vi "upload.list_parts.vi"(8 "error in":errorcluster, 11 "Multipart Upload":refnum<class "Multipart Upload.lvclass">) -> (0 "error out":errorcluster, 3 "Multipart Upload out":refnum<class "Multipart Upload.lvclass">)   [LabVIEW 2020, in "Multipart Upload.lvclass"]
doc: "Lists the parts that have been uploaded for a given uploadId."
uses:
  Multipart Upload.lvclass
  Multipart Upload.lvclass/Multipart Upload.ctl
  Nominal Client/Nominal Client.lvclass/Nominal Client.ctl
  72e5dcd8-64cf-4027-aada-cf32ea863567.vi
  nominal_client.get.vi
  parts.set.vi
  Nominal Client/create.authorization_header.vi
  Nominal Client/trace.payload_sent.vi
  Nominal Client/trace.payload_received.vi
  Nominal Client/error.vi
  Nominal Client/api_token.get.vi
  Nominal Client/error.vi/859f8e04-e495-489b-b5b4-7ac163f56130.vi
  submodules/reqwest-labview/lv-src/reqwest/get.vi
  <vilib>/JDP Science/JSONtext/Get all Object Items.vi
  <vilib>/Utility/error.llb/Error Cluster From Error Code.vi
  <vilib>/JDP Science/JSONtext/JSON text to Variant.vi
  Nominal Client/Nominal Client.lvclass
  <vilib>/JDP Science/JSONtext/LVClass Serializer/JSONtext LVClass Serializer.lvclass
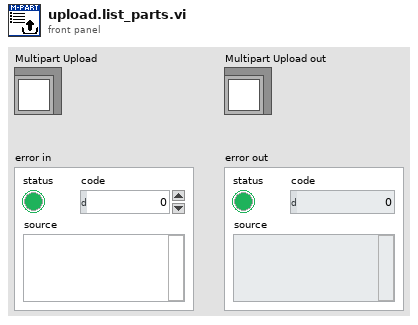
[diagram p1: front panel]
types:
  T1 = cluster{"partNumber":i32, "etag":string, "size":i32}[]
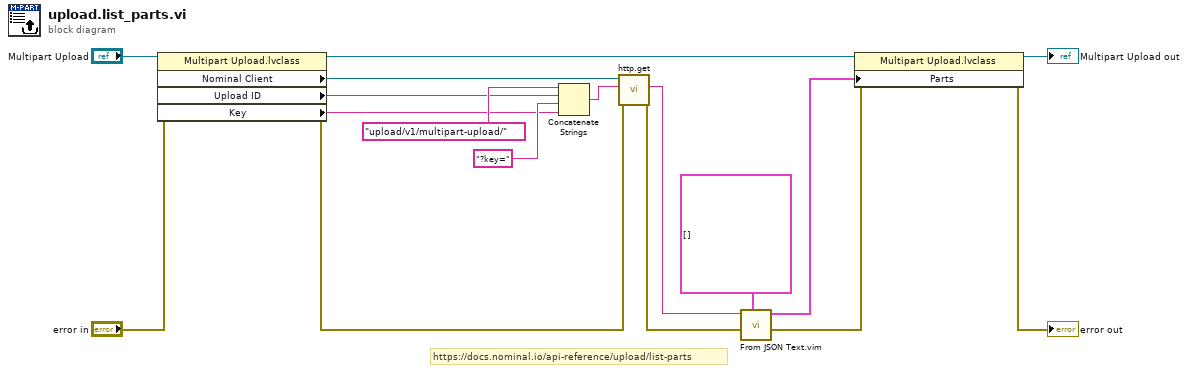
[diagram p0: block diagram]
diagram:
  # "https://docs.nominal.io/api-reference/upload/list-parts"
  n1 = property class="Multipart Upload.lvclass"(reference="Multipart Upload", error in="error in") -> (reference out=w7:refnum<class "Multipart Upload.lvclass">, error out=w9:errorcluster, "Nominal Client"=w2:refnum<class "Nominal Client.lvclass">, "Upload ID"=w11:string, "Key"=w10:string)
  n2 = Concatenate Strings("upload/v1/multipart-upload/", w11, "?key=", w10) -> (w15:string)
  n3 = call "http.get.vi"("error in"=w9, "Path"=w15, "Nominal Client in"=w2) -> ("error out"=w5:errorcluster, "Response"=w13:string)  [unwired: 6 in, 1 out]
  n4 = call "From JSON Text.vim"("Data Type and Default Value"=T1 [], "error in (no error)"=w5, "JSON"=w13) -> ("error out"=w3:errorcluster, "Data out"=w1:T1)  [unwired: 7 in]
  n5 = property class="Multipart Upload.lvclass"(reference=w7, error in=w3, "Parts"=w1) -> (reference out=→"Multipart Upload out":refnum<class "Multipart Upload.lvclass">, error out=→"error out":errorcluster)
